vi "Waka front panel.vi"() -> ()   [LabVIEW 2024]
uses:
  Helper/Key CAN statistics.ctl
  <instrlib>/KDI Digital Instrumentation/API_for_PCAN_BASIC_FD/TPCANHandle.ctl
  <instrlib>/KDI Digital Instrumentation/API_for_PCAN_BASIC_FD/TPCANBaudrate.ctl
  <vilib>/Utility/error.llb/DialogType.ctl
  <vilib>/Utility/sysdir.llb/System Directory Type.ctl
  <vilib>/Platform/TimedLoop/XDataNode/timing_clust.ctl
  <vilib>/Platform/TimedLoop/XDataNode/nitl_modes.ctl
  <vilib>/Platform/TimedLoop/XDataNode/wakeup.ctl
  ZeroJet Test Systems/Instruments/PCAN/Generate BCI frames.vi
  ZeroJet Test Systems/Production Data/TestStand Results/MEASUREMENT float.vi
  <instrlib>/IT6000C/Public/Configure/Source/Configure Voltage Positive Slew.vi
  <userlib>/ZeroJet/IT6000C/Set watchdog.vi
  ZeroJet Test Systems/Instruments/PCAN/Read can to signal maps.vi
  ZeroJet Test Systems/Production Data/TestStand Results/MEASUREMENT power spectrum.vi
  <vilib>/platform/TimedLoop/XDataNode/XDataNode.xnode
  ZeroJet Test Systems/Production Data/Production Data.lvlib
  <userlib>/ZeroJet/IT6000C/IT6000C production.lvlib
  <vilib>/Platform/TimedLoop/XDataNode/XDNodeRunTimeDep.lvlib
  ZeroJet Test Systems/Instruments/PCAN/PCan_Xnet.lvlib
  <instrlib>/IT6000C/IT6000C.lvlib
panel:
  in  "stop":bool
  out "Main selector":enum32{"Power supply Setup", "CAN Setup", "Run"}(tab)
  in  "IT6000C instrument address":refnum<visa-resource-name>="USB0::0x2EC7::0x6000::804050011767650001::INSTR"
  in  "Voltage rise time":dbl=5.0 format="%#_13gs"
  in  "Power supply watchdog time":dbl=2.0 min=0.0 max=10.0 step=0.1 format="%#_13gs"
  in  "Button - Connect power supply":bool
  in  "Button - Don't use power supply":bool
  out "LED - Supply connected":bool
  out "Connection response":string
  in  "Button - Power supply next":bool
  in  "Voltage":dbl=52.0 min=0.0 format="%.2fV"
  in  "Current":dbl=300.0 format="%#_gA"
  in  "Button - Power supply next":bool
  out "LED - Setting up CAN":bool
  out "CAN Status":string
  in  "Button - CAN data storage location":bool
  in  "Vibration capture time (s)":dbl=60.0
  in  "Test Runtime HH:MM":dbl=2700.0 format="%<%H:%M>t"
  in  "Batch Serial Number":string="RevC Pilot Run"
  in  "Part Number":string="RevC Jet Pump"
  in  "Serial Number":string
  in  "Button - Reset hour counter":bool
  in  "Button - Reset timer":bool
  out "Left spectrum channel":cluster{"f0":dbl, "df":dbl, "magnitude":dbl[]}(graph)
  out "Right spectrum channel":cluster{"f0":dbl, "df":dbl, "magnitude":dbl[]}(graph)
  in  "Run tab data":enum32{"Key Data", "All can data", "Errors"}(tab)
  out "Supply Voltage":dbl format="%.2g"
  out "Supply Current":dbl format="%.2g"
  out "Key statistics":T1
  out "Signal map":map{string, dbl}(c390)
  out "Error and warning map":map{string, i8}(c390)
  out "Can data write loop":errorcluster
  out "Power supply update loop":errorcluster
  out "Elapsed time loop":errorcluster
  out "Setup loop":errorcluster
  out "Spectrum loop":errorcluster
  out "Elapsed Time (s)":dbl format="%<%H:%M:%S>t"
  out "T-":dbl caption="Elapsed Time (s)" format="%<%H:%M:%S>t"
  # "Power supply setup"
  # "1. Click in this box and select the instrument address for the power supply\n\n\n\n2. Choose the voltage rise time and the watchdog time\n    - Default: 5s votlage rise time\n    - Default: 2s power supply watchdog time\nYou will likely not need to modify these numbers\n\n\n3. Click on connect or don't use power supply\n    - If you are using a battery, then select don't use"
  # "UUT Details"
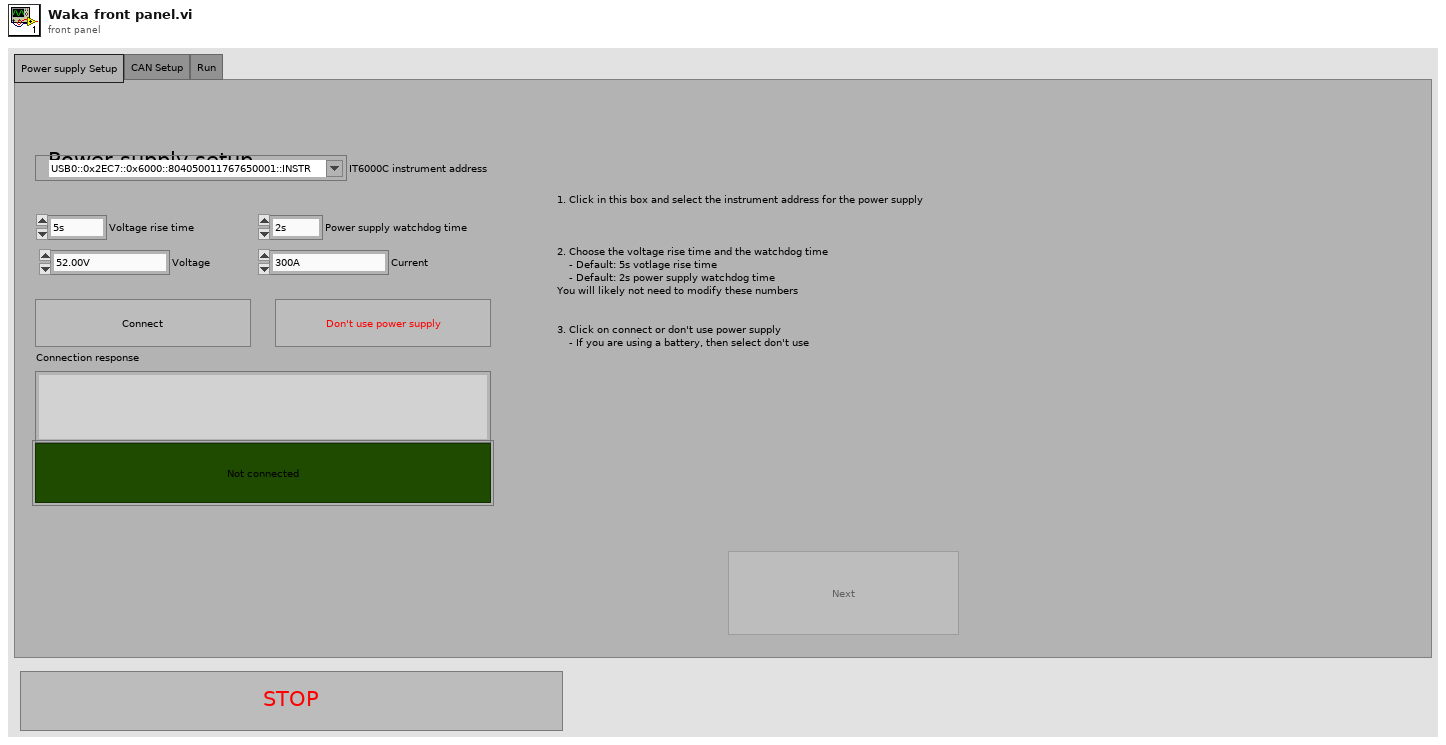
[diagram p1: front panel]
types:
  T1 = typedef "Key CAN statistics.ctl" = cluster{"Drive voltage ":dbl, "High current volt drop":dbl, "High current series resistance":dbl, "Drive phase amps":dbl, "Torque request":dbl, "Motor temp":dbl, "GPS Status":dbl, "RPM":dbl, "Capacitor temp":dbl, "MCM ID":dbl, "MCM Version":string}
  T2 = enum8{"Enabled", "Disabled", "Disabled and Grayed Out"}
  T3 = typedef "TPCANBaudrate.ctl" = enum16{"PCAN_BAUD_1M 0x0014", "PCAN_BAUD_800K 0x0016", "PCAN_BAUD_500K 0x001C", "PCAN_BAUD_250K 0x011C", "PCAN_BAUD_125K 0x031C", "PCAN_BAUD_100K 0x432F", "PCAN_BAUD_95K 0xC34E", "PCAN_BAUD_83K 0x852B", "PCAN_BAUD_50K 0x472F", "PCAN_BAUD_47K 0x1414", "PCAN_BAUD_33K 0x8B2F", "PCAN_BAUD_20K 0x532F", "PCAN_BAUD_10K 0x672F", "PCAN_BAUD_5K 0x7F7F", "User Baudrate"}
  T4 = typedef "TPCANHandle.ctl" = enum16{"PCAN_NONEBUS  0x000", "PCAN_ISABUS1  0x21", "PCAN_ISABUS2  0x22", "PCAN_ISABUS3  0x23", "PCAN_ISABUS4  0x24", "PCAN_ISABUS5  0x25", "PCAN_ISABUS6  0x26", "PCAN_ISABUS7  0x27", "PCAN_ISABUS8  0x28", "PCAN_DNGBUS1  0x31", "PCAN_PCIBUS1  0x41", "PCAN_PCIBUS1  0x42", "PCAN_PCIBUS1  0x43", "PCAN_PCIBUS1  0x44", "PCAN_PCIBUS1  0x45", "PCAN_PCIBUS1  0x46", "PCAN_PCIBUS1  0x47", "PCAN_PCIBUS1  0x48", "PCAN_PCIBUS1  0x409", "PCAN_PCIBUS1  0x40A", "PCAN_PCIBUS1  0x40B", "PCAN_PCIBUS1  0x40C", "PCAN_PCIBUS1  0x40D", "PCAN_PCIBUS1  0x40E", "PCAN_PCIBUS1  0x40F", "PCAN_PCIBUS1  0x410", "PCAN_USBBUS1  0x51", "PCAN_USBBUS2  0x52", "PCAN_USBBUS3  0x53", "PCAN_USBBUS4  0x54", "PCAN_USBBUS5  0x55", "PCAN_USBBUS6  0x56", "PCAN_USBBUS7  0x57", "PCAN_USBBUS8  0x58", "PCAN_USBBUS9  0x509", "PCAN_USBBUS10  0x50A", "PCAN_USBBUS11  0x50B", "PCAN_USBBUS12  0x50C", "PCAN_USBBUS13  0x50D", "PCAN_USBBUS14  0x50E", "PCAN_USBBUS15  0x50F", "PCAN_USBBUS16  0x510", "PCAN_PCCBUS1  0x61", "PCAN_PCCBUS2  0x62", "PCAN_LANBUS1  0x801", "PCAN_LANBUS2  0x802", "PCAN_LANBUS3  0x803", "PCAN_LANBUS4  0x804", "PCAN_LANBUS5  0x805", "PCAN_LANBUS6  0x806", "PCAN_LANBUS7  0x807", "PCAN_LANBUS8  0x808", "PCAN_LANBUS9  0x809", "PCAN_LANBUS10  0x80A", "PCAN_LANBUS11  0x80B", "PCAN_LANBUS12  0x80C", "PCAN_LANBUS13  0x80D", "PCAN_LANBUS14  0x80E", "PCAN_LANBUS15  0x80F", "PCAN_LANBUS16  0x810"}
  T5 = typedef "DialogType.ctl" = u16
  T6 = typedef "NI_Database_API.lvlib/Conn ObjectReference.ctl" = refnum<k1>
  T7 = typedef "System Directory Type.ctl" = i32
  T8 = enum16{"open", "open or create", "create or replace", "create", "open (read-only)"}
  T9 = typedef "XDNodeRunTimeDep.lvlib/timing_clust.ctl" = cluster{"Expected End [f-1]":u64, "Actual End [f-1]":u64, "Finished Late? [f-1]":bool, "Expected End [i-1]":u64, "Actual End [i-1]":u64, "Finished Late? [i-1]":bool, "Expected Start [i]":u64, "Actual Start [i]":u64, "Expected Start [f]":u64, "Actual Start [f]":u64, "Source Name":string, "Structure Name":string, "Period":i64, "Deadline":i64, "Offset":i64, "Start":i64, "Priority":i32, "Timeout":i32, "Mode":T10, "Wakeup Reason":T11, "Error":errorcluster, "Source Type":string, "Secondary Source Type":string, "Global End Time":u64, "Global Start Time":u64, "Frame Duration":u64, "Iteration Duration":u64, "Assigned CPU":i32, "I/O Scan Engine Mode":u32}
  T10 = typedef "XDNodeRunTimeDep.lvlib/nitl_modes.ctl" = enum32{"No Change", "Process missed periods, maintain original phase", "Discard missed periods, maintain original phase", "Process missed periods, ignore original phase", "Discard missed periods, ignore original phase"}
  T11 = typedef "XDNodeRunTimeDep.lvlib/wakeup.ctl" = enum32{"Normal", "Aborted", "Asynchronous wakeup", "Timing source error", "Timed loop error", "Timeout"}
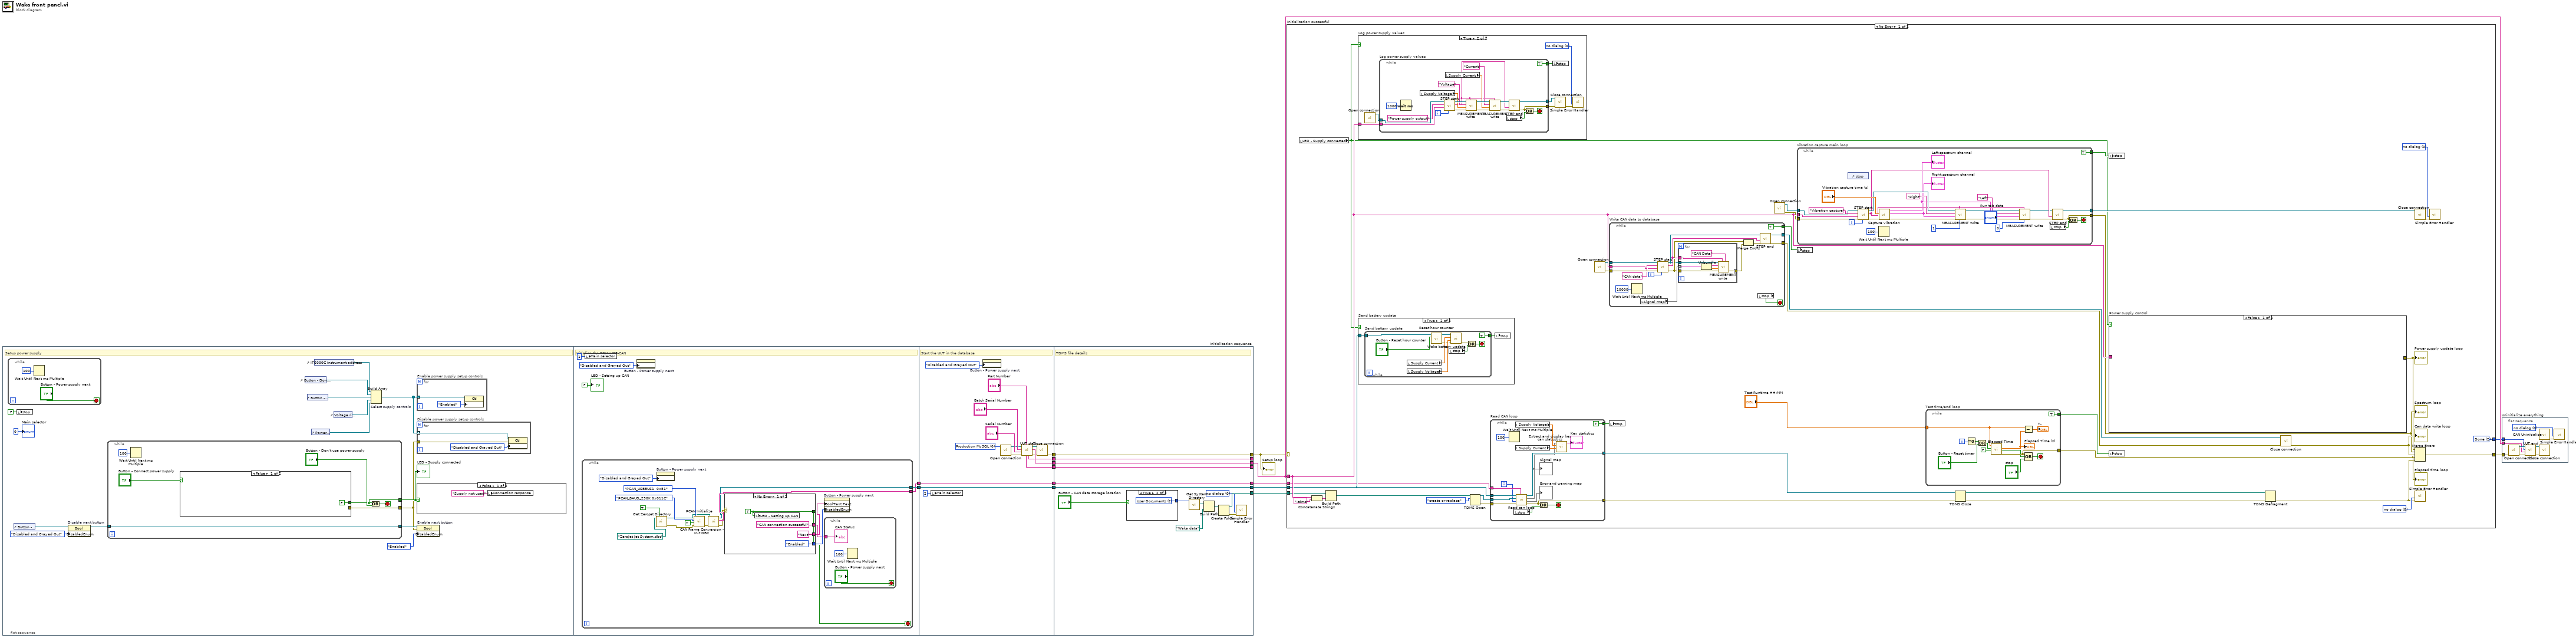
[diagram p0: block diagram]
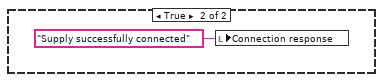
[diagram p2: hidden frame]
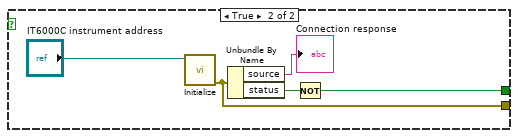
[diagram p3: hidden frame]
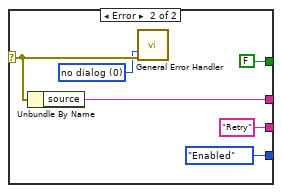
[diagram p4: hidden frame]
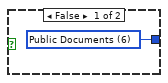
[diagram p5: hidden frame]
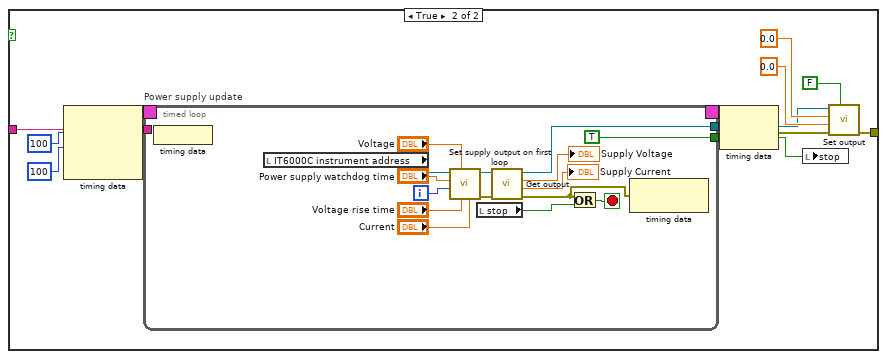
[diagram p7: hidden frame]
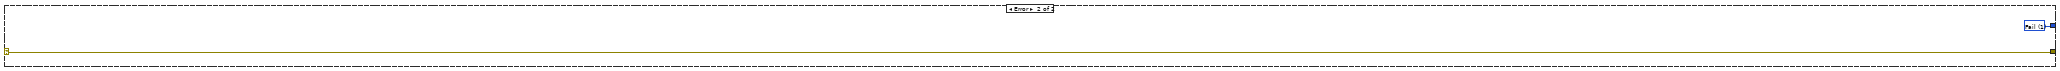
[diagram p9: hidden frame]
diagram:
  n1 = flat-sequence "Initialization sequence" {
    tunnel: [w55] -> w13
    tunnel: [w54] -> w12
    tunnel: w13 -> [w89]
    tunnel: w12 -> [w88]
    tunnel: [w102] -> w9
    tunnel: [w101] -> w8
    tunnel: [w100] -> w7
    tunnel: [w92] -> w6
    tunnel: [w89] -> w5
    tunnel: [w88] -> w4
    tunnel: [w112] -> w10
    tunnel: [w113] -> w11
    tunnel: [w105] -> w2
    tunnel: [w114] -> _
    tunnel: [w115] -> _
    tunnel: [w116] -> w15
    tunnel: w9 -> [w116]
    tunnel: w8 -> [w115]
    tunnel: w7 -> [w114]
    tunnel: w6 -> [w105]
    tunnel: w5 -> [w113]
    tunnel: w4 -> [w112]
    tunnel: [w108] -> w3
    frame #0 {
      # "Setup power supply"
      n2 = while {
        stop <- "Button - Power supply next" stop-if-true
        n3 = Wait Until Next ms Multiple(millisecond multiple=u32 100) -> ()  [unwired: 1 out]
      }
      n4 = control-ref of="Button - Power supply next"() -> (w24:refnum<vi>)
      n5 = local write "stop"(FALSE ("Release all channels first")) -> ()
      n6 = property on="Disable next button" class="Bool"(reference=w24, "DisabledEnum"=T2."Disabled and Grayed Out" ("Disabled")) -> (reference out=w21:refnum<vi>)  [unwired: 1 in, 1 out]
      n7 = while {
        tunnel: [w43] -> w19
        tunnel: [w42] -> w22
        tunnel: w21 -> [w42]
        tunnel: [w41] -> w17
        stop <- w44 stop-if-true
        n8 = Wait Until Next ms Multiple(millisecond multiple=u32 100) -> ()  [unwired: 1 out]
        n9 = case shown="False" "Button - Connect power supply" {
          tunnel: [FALSE w50] -> w43
          tunnel: [_ w48] -> w41
          frame False {
          }
          frame True {
            n10 = call <instrlib>:"Initialize.vi"("VISA resource name"="IT6000C instrument address") -> ("error out"=w48:errorcluster)  [unwired: 9 in, 1 out]
            n11 = Unbundle By Name(w48) -> ("source"=→"Connection response":string, "status"=w51:bool)
            n12 = Not(x=w51) -> (.not. x?=w50:bool)
          }
        }
        n13 = Or(x=w43, y="Button - Don't use power supply") -> (x .or. y?=w44:bool)
      }
      "LED - Supply connected" <- w19
      n14 = control-ref of="Button - Don't use power supply"() -> (w29:refnum<vi>)
      n15 = control-ref of="Button - Connect power supply"() -> (w28:refnum<vi>)
      n16 = control-ref of="Power supply watchdog time"() -> (w26:refnum<vi>)
      n17 = control-ref of="IT6000C instrument address"() -> (w30:refnum<vi>)
      n18 = control-ref of="Voltage rise time"() -> (w27:refnum<vi>)
      n19 = Build Array "Select supply controls"(w30, w29, w28, w27, w26) -> (w16:refnum<vi>[])
      n20 = for "Enable power supply setup controls" {
        tunnel: w16 -> [w35] mode=indexing
        n21 = property class="Ctl"(reference=w35, "DisabledEnum"=T2."Enabled" ("Disabled")) -> ()  [unwired: 1 in, 2 out]
      }
      n22 = for "Disable power supply setup controls" {
        tunnel: w16 -> [w33] mode=indexing
        tunnel: w17 -> [w31]
        n23 = property class="Ctl"(reference=w33, error in=w31, "DisabledEnum"=T2."Disabled and Grayed Out" ("Disabled")) -> ()  [unwired: 2 out]
      }
      n24 = case "Update connection response" shown="False" w19 {
        frame False {
          n25 = local write "Connection response"("Supply not used" ("Connection response")) -> ()
        }
        frame True {
          n26 = local write "Connection response"("Supply successfully connected" ("Connection response")) -> ()
        }
      }
      n27 = property on="Enable next button" class="Bool"(reference=w22, error in=w17, "DisabledEnum"=T2."Enabled" ("Disabled")) -> ()  [unwired: 2 out]
      "Main selector" <- 0
    }
    frame #1 {
      # "Initialise the PCAN USB-CAN"
      n28 = while {
        tunnel: [w69] -> w54
        tunnel: [w68] -> w55
        stop <- w60 stop-if-true
        n29 = call "Get ZeroJet Directory.vi"("Expect file to be present"=TRUE, "Data directory subpath"=path "ZeroJet Jet System.dbc") -> ("error out"=w65:errorcluster, "appended path"=w66:path)  [unwired: 7 in, 1 out]
        n30 = property on="Button - Power supply next" class="Bool"("DisabledEnum"=T2."Disabled and Grayed Out" ("Disabled")) -> ()  [unwired: 2 in, 2 out]
        n31 = call "PCAN Initialize.vi"("error in"=w65, "Release all channels first"=TRUE, "TPCANBaudrate"=TPCANBaudrate."PCAN_BAUD_250K 0x011C", "TPCANHandle"=TPCANHandle."PCAN_USBBUS1  0x51") -> ("error out"=w70:errorcluster)  [unwired: 6 in, 1 out]
        n32 = call "CAN Frame Conversion - Init DBC.vi"("error in (no error)"=w70, "DBC Path"=w66) -> ("error out"=w64:errorcluster, "Signals For Conversion"=w69:string[], "Frame Signal Conversion out"=w68:refnum<class "Frame Signal Conversion.lvclass">)  [unwired: 7 in]
        n33 = case shown="No Error" w64 {
          selector: w64 -> [_ w79]
          tunnel: ["Next" ("Boolean Text.Text") "Retry" ("Boolean Text.Text")] -> w62
          tunnel: [T2."Enabled" ("Disabled") T2."Enabled" ("Disabled")] -> w61
          tunnel: ["CAN connection successful" ("source") w81] -> w59
          tunnel: [w74 FALSE ("LED - Setting up CAN")] -> w60
          frame No Error {
            w74 = TRUE ("LED - Setting up CAN")
            n34 = local write "LED - Setting up CAN"(w74) -> ()
          }
          frame Error {
            w78 = T5 0 items=["no dialog", "OK message", "continue or stop message", "OK message + warnings", "continue/stop + warnings"] ("type of dialog (OK msg:1)")
            n35 = Unbundle By Name(w79) -> ("source"=w81:string)
            n36 = call <vilib>:"General Error Handler.vi"("type of dialog (OK msg:1)"=w78, "error in (no error)"=w79) -> ()  [unwired: 9 in, 5 out]
          }
        }
        n37 = property on="Button - Power supply next" class="Bool"("BoolText.Text"=w62, "DisabledEnum"=w61) -> ()  [unwired: 2 in, 2 out]
        n38 = while {
          tunnel: w59 -> [w85]
          stop <- "Button - Power supply next" stop-if-true
          n39 = Wait Until Next ms Multiple(millisecond multiple=u32 100) -> ()  [unwired: 1 out]
          "CAN Status" <- w85
        }
      }
      n40 = local write "Main selector"(1) -> ()
      n41 = property on="Button - Power supply next" class="Bool"("DisabledEnum"=T2."Disabled and Grayed Out" ("Disabled")) -> ()  [unwired: 2 in, 2 out]
      "LED - Setting up CAN" <- FALSE
    }
    frame #2 {
      w91 = u16 0 items=["Production MySQL"] ("Database")
      # "Start the UUT in the database"
      n42 = local write "Main selector"(2) -> ()
      n43 = property on="Button - Power supply next" class="Bool"("DisabledEnum"=T2."Disabled and Grayed Out" ("Disabled")) -> ()  [unwired: 2 in, 2 out]
      n44 = call "Open connection.vi"("Database"=w91) -> ("error out"=w95:errorcluster, "connection reference"=w97:T6)  [unwired: 9 in]
      n45 = call "UUT start.vi"("Part Number"="Part Number", "error in (no error)"=w95, "Serial Number"="Serial Number", "Batch Serial Number"="Batch Serial Number", "connection reference"=w97) -> ("error out"=w93:errorcluster, "UUT GUID"=w102:string, "connection reference out"=w94:T6, "Username"=w101:string, "Station name"=w100:string)  [unwired: 2 in]
      n46 = call "Close connection.vi"("error in"=w93, "connection reference"=w94) -> ("error out"=w92:errorcluster)  [unwired: 9 in]
    }
    frame #3 {
      w103 = T5 0 items=["no dialog", "OK message", "continue or stop message", "OK message + warnings", "continue/stop + warnings"] ("type of dialog (OK msg:1)")
      # "TDMS file details"
      n47 = case shown="True" "Button - CAN data storage location" {
        tunnel: [w117 w118] -> w107
        frame False {
          w117 = T7 6 items=["User Home"=0, "User Desktop"=1, "User Documents"=2, "User Application Data"=3, "User Preferences"=4, "User Temporary"=5, "Public Documents"=6, "Public Application Data"=7, "Public Preferences"=8, "Public Cache"=13, "System Core Libraries"=9, "System Installed Libraries"=10, "Application Files"=11, "Boot Volume Root"=12] ("system directory type")
        }
        frame True {
          w118 = T7 2 items=["User Home"=0, "User Desktop"=1, "User Documents"=2, "User Application Data"=3, "User Preferences"=4, "User Temporary"=5, "Public Documents"=6, "Public Application Data"=7, "Public Preferences"=8, "Public Cache"=13, "System Core Libraries"=9, "System Installed Libraries"=10, "Application Files"=11, "Boot Volume Root"=12] ("system directory type")
        }
      }
      n48 = call <vilib>:"Get System Directory.vi"("system directory type"=w107) -> ("system directory"=w111:path)  [unwired: 10 in]
      n49 = Build Path(base path=w111, name or relative path=path "Waka data") -> (appended path=w109:path)
      n50 = Create Folder(path (use dialog)=w109) -> (created path=w108:path, error out=w104:errorcluster)  [unwired: 2 in, 1 out]
      n51 = call <vilib>:"Simple Error Handler.vi"("type of dialog (OK msg:1)"=w103, "error in (no error)"=w104) -> ()  [unwired: 3 in, 5 out]
    }
  }
  n52 = case "Initialization successful" shown="No Error" w2 {
    selector: w2 -> [_ w312]
    tunnel: w15 -> [w152 _]
    tunnel: [w155 w313] -> w14
    tunnel: w11 -> [w147 _]
    tunnel: w10 -> [w146 _]
    tunnel: w3 -> [w148 _]
    tunnel: [w124 w312] -> w1
    frame No Error {
      w139 = T5 0 items=["no dialog", "OK message", "continue or stop message", "OK message + warnings", "continue/stop + warnings"] ("type of dialog (OK msg:1)")
      w142 = T5 0 items=["no dialog", "OK message", "continue or stop message", "OK message + warnings", "continue/stop + warnings"] ("type of dialog (OK msg:1)")
      w155 = u16 2 items=["Pass", "Fail", "Done", "Error"] ("Test Result")
      n53 = local read "LED - Supply connected"() -> (w149:bool)
      n54 = Concatenate Strings(w152, ".tdms" ("string")) -> (w127:string)
      n55 = Build Path(base path=w148, name or relative path=w127) -> (appended path=w126:path)
      n56 = case "Log power supply values" shown="True" w149 {
        tunnel: w152 -> [_ w159]
        frame False {
        }
        frame True {
          w158 = T5 0 items=["no dialog", "OK message", "continue or stop message", "OK message + warnings", "continue/stop + warnings"] ("type of dialog (OK msg:1)")
          n57 = call "Open connection.vi"() -> ("connection reference"=w157:T6)  [unwired: 10 in, 1 out]
          n58 = while "Log power supply values" {
            tunnel: w157 -> [w183]
            tunnel: w159 -> [w175]
            tunnel: [w168] -> w156
            tunnel: [w164] -> w160
            tunnel: [TRUE] -> w162
            i -> [w166]
            stop <- w169 stop-if-true
            n59 = Wait (ms)(milliseconds to wait=u32 1000) -> ()  [unwired: 1 out]
            n60 = local read "Supply Voltage"() -> (w178:dbl)
            n61 = call "STEP start.vi"("Loop index"=w166, "UUT GUID"=w175, "Step name"="Power supply output" ("Step category"), "connection reference"=w183) -> ("error out"=w173:errorcluster, "Step GUID"=w174:string, "connection reference out"=w182:T6)  [unwired: 5 in]
            n62 = local read "Supply Current"() -> (w179:dbl)
            n63 = call-poly "MEASUREMENT write.vi"("Step Parent GUID"=w174, "error in (no error)"=w173, "Input data"=w178, "Step name"="Voltage", "connection reference"=w182) -> ("error out"=w172:errorcluster, "connection reference out"=w181:T6)  [unwired: 4 in, 1 out]
            n64 = call-poly "MEASUREMENT write.vi"("Step Parent GUID"=w174, "error in (no error)"=w172, "Input data"=w179, "Step name"="Current", "connection reference"=w181) -> ("error out"=w171:errorcluster, "connection reference out"=w180:T6)  [unwired: 4 in, 1 out]
            n65 = local read "stop"() -> (w170:bool)
            n66 = call "STEP end.vi"("error in (no error)"=w171, "Step GUID"=w174, "connection reference"=w180) -> ("error out"=w168:errorcluster, "connection reference out"=w164:T6)  [unwired: 7 in]
            n67 = Or(x=w168, y=w170) -> (x .or. y?=w169:bool)
          }
          n68 = local write "stop"(w162) -> ()
          n69 = call "Close connection.vi"("error in"=w156, "connection reference"=w160) -> ("error out"=w161:errorcluster)  [unwired: 9 in]
          n70 = call <vilib>:"Simple Error Handler.vi"("type of dialog (OK msg:1)"=w158, "error in (no error)"=w161) -> ()  [unwired: 3 in, 5 out]
        }
      }
      n71 = case "Send battery update" shown="True" w149 {
        tunnel: w147 -> [_ w222]
        frame False {
        }
        frame True {
          n72 = while "Send battery update" {
            tunnel: w222 -> [w225]
            tunnel: [TRUE] -> w221
            stop <- w231 stop-if-true
            n73 = local read "Supply Current"() -> (w228:dbl)
            n74 = local read "Supply Voltage"() -> (w227:dbl)
            n75 = call "Reset hour counter.vi"("Button - Reset hour counter"="Button - Reset hour counter", "Frame Signal Conversion in"=w225) -> ("error out"=w223:errorcluster, "Frame Signal Conversion out"=w224:refnum<class "Frame Signal Conversion.lvclass">)  [unwired: 8 in]
            n76 = local read "stop"() -> (w232:bool)
            n77 = call "Waka battery update.vi"("error in (no error)"=w223, "Supply Voltage"=w227, "Supply Current"=w228, "Frame Signal Conversion in"=w224) -> ("error out"=w230:errorcluster)  [unwired: 7 in]
            n78 = Or(x=w230, y=w232) -> (x .or. y?=w231:bool)
          }
          n79 = local write "stop"(w221) -> ()
        }
      }
      n80 = TDMS Open(10:T8."create or replace" ("operation (0:open)"), 11:w126) -> (0:w141:errorcluster, 3:w140:refnum<k34>)  [unwired: 5 in]
      n81 = while "Read CAN loop" {
        tunnel: w147 -> [w265]
        tunnel: w146 -> [w264]
        tunnel: [w258] -> w125
        tunnel: [TRUE ("stop")] -> w135
        tunnel: w141 -> [w259]
        tunnel: w140 -> [w261]
        tunnel: [w262] -> w138
        i -> [w260]
        stop <- w271 stop-if-true
        n82 = Wait Until Next ms Multiple(millisecond multiple=u32 100) -> ()  [unwired: 1 out]
        n83 = local read "stop"() -> (w270:bool)
        n84 = local read "Supply Voltage"() -> (w268:dbl)
        n85 = local read "Supply Current"() -> (w267:dbl)
        n86 = call "Read can loop.vi"("Signals For Conversion"=w264, "error in (no error)"=w259, "Numeric"=w260, "tdms file in"=w261, "Frame Signal Conversion in"=w265) -> ("error out"=w258:errorcluster, "Error and warning map"=→"Error and warning map":map{string, i8}, "Signal map"=w257:map{string, dbl}, "tdms file out"=w262:refnum<k34>)  [unwired: 3 in]
        "Signal map" <- w257
        n87 = Or(x=w258, y=w270) -> (x .or. y?=w271:bool)
        n88 = call "Extract and display key can statisctics.vi"("Supply current output"=w267, "Supply voltage output"=w268, "Signal map in"=w257) -> ("Key statistics"=→"Key statistics":T1)  [unwired: 8 in]
      }
      n89 = call "Open connection.vi"() -> ("error out"=w131:errorcluster, "connection reference"=w133:T6)  [unwired: 10 in]
      n90 = while "Write CAN data to database" {
        tunnel: [TRUE] -> w134
        tunnel: w133 -> [w244]
        tunnel: [w243] -> w132
        tunnel: w131 -> [w242]
        tunnel: [w239] -> w130
        tunnel: w152 -> [w236]
        i -> [w235]
        stop <- w247 stop-if-true
        n91 = Wait Until Next ms Multiple(millisecond multiple=u32 10000) -> ()  [unwired: 1 out]
        n92 = local read "Signal map"() -> (w245:map{string, dbl})
        n93 = call "STEP start.vi"("Loop index"=w235, "error in (no error)"=w242, "UUT GUID"=w236, "Step name"="CAN data", "connection reference"=w244) -> ("error out"=w234:errorcluster, "Step GUID"=w238:string, "connection reference out"=w233:T6)  [unwired: 4 in]
        n94 = for {
          tunnel: w233 -> [w256]
          tunnel: w245 -> [w255] mode=indexing
          tunnel: w238 -> [w252]
          tunnel: w234 -> [w250]
          tunnel: [w249] -> w241 mode=indexing
          n95 = Unbundle(w255) -> (w254:string, w253:dbl)
          n96 = call-poly "MEASUREMENT write.vi"("Step category"="CAN Data", "Step Parent GUID"=w252, "error in (no error)"=w250, "Input data"=w253, "Step name"=w254, "connection reference"=w256) -> ("error out"=w249:errorcluster)  [unwired: 3 in, 2 out]
        }
        n97 = Merge Errors(w234, w241) -> (w240:errorcluster)
        n98 = local read "stop"() -> (w247:bool)
        n99 = call "STEP end.vi"("error in (no error)"=w240, "Step GUID"=w238, "connection reference"=w233) -> ("error out"=w239:errorcluster, "connection reference out"=w243:T6)  [unwired: 7 in]
      }
      n100 = local write "stop"(w135) -> ()
      n101 = call "Open connection.vi"() -> ("error out"=w144:errorcluster, "connection reference"=w145:T6)  [unwired: 10 in]
      n102 = while "Vibration capture main loop" {
        tunnel: w152 -> [w294]
        tunnel: [w284] -> w154
        tunnel: [w277] -> w120
        tunnel: [TRUE] -> w153
        tunnel: w145 -> [w275]
        tunnel: w144 -> [w274]
        i -> [w283]
        stop <- w297 stop-if-true
        n103 = control-ref of="stop"() -> ()  [unwired: 1 out]
        n104 = call "STEP start.vi"("Loop index"=w283, "error in (no error)"=w274, "UUT GUID"=w294, "Step name"="Vibration capture", "connection reference"=w275) -> ("error out"=w293:errorcluster, "Step GUID"=w286:string, "connection reference out"=w292:T6)  [unwired: 4 in]
        n105 = Wait Until Next ms Multiple(millisecond multiple=u32 100) -> ()  [unwired: 1 out]
        n106 = call "Capture vibration.vi"("error in (no error)"=w293, "Vibration capture time (s)"="Vibration capture time (s)") -> ("error out"=w278:errorcluster, "Frequency power spectrum"=w279:cluster{"f0":dbl, "df":dbl, "magnitude":dbl[]}, "Frequency power spectrum 2"=w280:cluster{"f0":dbl, "df":dbl, "magnitude":dbl[]})  [unwired: 7 in]
        "Left spectrum channel" <- w280
        "Right spectrum channel" <- w279
        n107 = call-poly "MEASUREMENT write.vi"("Order number"=1, "Step GUID"=w286, "error in (no error)"=w278, "Input frequency power spectrum"=w279, "Step name"="Right", "connection reference"=w292) -> ("error out"=w291:errorcluster, "connection reference out"=w290:T6)  [unwired: 3 in, 1 out]
        n108 = call-poly "MEASUREMENT write.vi"("Order number"=0, "Step GUID"=w286, "error in (no error)"=w291, "Input frequency power spectrum"=w280, "Step name"="Left", "connection reference"=w290) -> ("error out"=w287:errorcluster, "connection reference out"=w285:T6)  [unwired: 3 in, 1 out]
        n109 = local read "stop"() -> (w296:bool)
        n110 = call "STEP end.vi"("error in (no error)"=w287, "Step GUID"=w286, "connection reference"=w285) -> ("error out"=w277:errorcluster, "connection reference out"=w284:T6)  [unwired: 7 in]
        n111 = Or(x=w277, y=w296) -> (x .or. y?=w297:bool)
      }
      "Spectrum loop" <- w120
      n112 = local write "stop"(w134) -> ()
      n113 = while "Test time/end loop" {
        tunnel: "Test Runtime HH:MM" -> [w307]
        tunnel: [TRUE] -> w150
        tunnel: [w302] -> w122
        i -> [w306]
        stop <- w299 stop-if-true
        n114 = Equal To 0?(x=w306) -> (x = 0?=w308:bool)
        n115 = Or(x=w308, y="Button - Reset timer") -> (x .or. y?=w304:bool)
        n116 = call "Elapsed Time"("Time Target (s)"=w307, "Reset"=w304, "Auto Reset"=FALSE) -> ("Elapsed Time (s)"=w311:dbl, "Time has Elapsed"=w301:bool, "error out"=w302:errorcluster)  [unwired: 9 in, 5 out]
        "Elapsed Time (s)" <- w311
        n117 = Subtract(x=w307, y=w311) -> (x-y=→"T-":dbl)
        n118 = Compound Arithmetic op=OR(w302, w301, "stop") -> (w299:bool)
      }
      "Elapsed time loop" <- w122
      n119 = TDMS Close(8:w125, 11:w138) -> (0:w136:errorcluster, 3:w137:path)
      n120 = local write "stop"(w153) -> ()
      n121 = case "Power supply control" shown="False" w149 {
        tunnel: w152 -> [_ w193]
        tunnel: [_ w184] -> w119
        frame False {
        }
        frame True {
          n122 = node-c288(i64 100 ("Period"), 100 ("Priority")) -> (w195:T9)  [unwired: 1 in]
          n123 = timed-loop "Power supply update" {
            tunnel: w193 -> [_]
            tunnel: [TRUE] -> w185
            timing: w195 -> [_]
            timing-out: [_] -> w194
            tunnel: [w204] -> w189
            i -> [w202]
            stop <- w200 stop-if-true
            n124 = node-c288() -> ()  [unwired: 1 in]
            n125 = local read "IT6000C instrument address"() -> (w205:refnum<visa-resource-name>)
            n126 = call "Set supply output on first loop.vi"("Current"="Current", "Voltage rise time"="Voltage rise time", "Voltage"="Voltage", "Numeric"=w202, "Power supply watchdog time"="Power supply watchdog time", "VISA Refnum in"=w205) -> ("error out"=w209:errorcluster, "VISA Refnum out"=w210:refnum<visa-resource-name>)  [unwired: 4 in]
            n127 = local read "stop"() -> (w201:bool)
            n128 = call <userlib>:"Get output.vi"("error in"=w209, "VISA resource name"=w210) -> ("error out"=w203:errorcluster, "Actual Current Level (A)"=→"Supply Current":dbl, "Actual Voltage Level (V)"=→"Supply Voltage":dbl, "VISA resource name out"=w204:refnum<visa-resource-name>)  [unwired: 6 in]
            n129 = Or(x=w203, y=w201) -> (x .or. y?=w200:bool)
            n130 = node-c288(w203) -> ()  [unwired: 1 out]
          }
          n131 = node-c288(w194) -> (w188:errorcluster)
          n132 = local write "stop"(w185) -> ()
          n133 = call <userlib>:"Set output.vi"("Output state"=FALSE, "error in"=w188, "Current(A)"=0.0, "Voltage(V)"=0.0, "VISA resource name"=w189) -> ("error out"=w184:errorcluster)  [unwired: 5 in, 1 out]
        }
      }
      "Power supply update loop" <- w119
      n134 = local write "stop"(w150) -> ()
      n135 = TDMS Defragment(4:w136, 7:w137) -> (0:w123:errorcluster)
      n136 = call "Close connection.vi"("error in"=w130, "connection reference"=w132) -> ("error out"=w121:errorcluster)  [unwired: 9 in]
      "Can data write loop" <- w121
      n137 = call "Close connection.vi"("connection reference"=w154) -> ("error out"=w143:errorcluster)  [unwired: 10 in]
      n138 = Merge Errors(w119, w120, w121, w122, w123) -> (w124:errorcluster)
      n139 = call <vilib>:"Simple Error Handler.vi"("type of dialog (OK msg:1)"=w139, "error in (no error)"=w123) -> ()  [unwired: 3 in, 5 out]
      n140 = call <vilib>:"Simple Error Handler.vi"("type of dialog (OK msg:1)"=w142, "error in (no error)"=w143) -> ()  [unwired: 3 in, 5 out]
    }
    frame Error {
      w313 = u16 1 items=["Pass", "Fail", "Done", "Error"] ("Test Result")
    }
  }
  n141 = flat-sequence "Uninitialize everything" {
    tunnel: w15 -> [w316]
    tunnel: w14 -> [w315]
    tunnel: w1 -> [w314]
    frame #0 {
      w321 = T5 0 items=["no dialog", "OK message", "continue or stop message", "OK message + warnings", "continue/stop + warnings"] ("type of dialog (OK msg:1)")
      n142 = call "Open connection.vi"("error in"=w314) -> ("error out"=w319:errorcluster, "connection reference"=w320:T6)  [unwired: 9 in]
      n143 = call "UUT end.vi"("error in (no error)"=w319, "Test UUID"=w316, "Test Result"=w315, "connection reference"=w320) -> ("error out"=w317:errorcluster, "connection reference out"=w318:T6)  [unwired: 6 in]
      n144 = call <instrlib>:"CAN Uninitialize.vi"() -> ("error out"=w322:errorcluster)  [unwired: 9 in, 2 out]
      n145 = call "Close connection.vi"("error in"=w317, "connection reference"=w318) -> ()  [unwired: 9 in, 1 out]
      n146 = call <vilib>:"Simple Error Handler.vi"("type of dialog (OK msg:1)"=w321, "error in (no error)"=w322) -> ()  [unwired: 3 in, 5 out]
    }
  }
  "Setup loop" <- w2
